vi "TransmissionAndAbsorptionSubVI.vi"(2 "FILTER":dbl[](array[numeric]), 3 "Stop REF":refnum<vi>, 4 "LED":dbl[](array[numeric])) -> (0 "Transmission":dbl[](array[numeric]), 1 "Absorption":dbl[](array[numeric]))   [LabVIEW 2021]
panel:
  in  "stop":bool
  in  "Array 2":dbl[](array[numeric])
  in  "Array":dbl[](array[numeric])
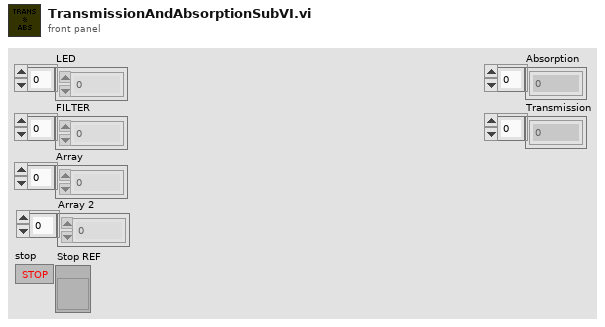
[diagram p1: front panel]
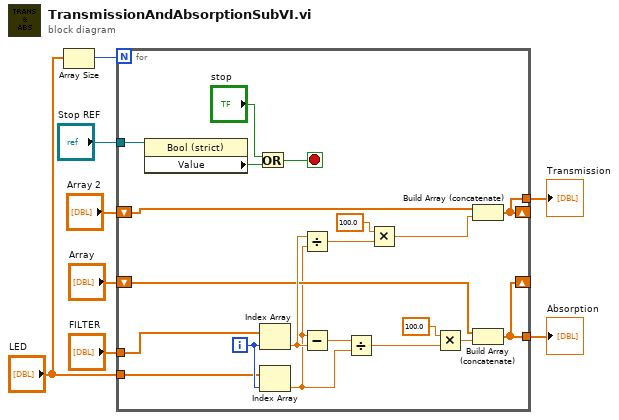
[diagram p0: block diagram]
diagram:
  n1 = Array Size(array="LED") -> (size(s)=w8:i32)
  n2 = for {
    N: w8 -> [_]
    tunnel: "LED" -> [w27]
    tunnel: "FILTER" -> [w26]
    shift-right: [w21] -> _
    shift-left: "Array 2" -> [w25]
    shift-right: [w22] -> _
    shift-left: "Array" -> [w23]
    tunnel: [w22] -> w5
    tunnel: [w21] -> w4
    tunnel: "Stop REF" -> [w16]
    i -> [w28]
    stop <- w17 stop-if-true
    n3 = property class="Bool (strict)"(reference=w16) -> ("Value"=w15:bool)  [unwired: 1 in, 2 out]
    n4 = Or(x="stop", y=w15) -> (x .or. y?=w17:bool)
    n5 = Index Array(array=w26, index=w28) -> (element=w24:dbl)
    n6 = Index Array(array=w27, index=w28) -> (element=w19:dbl)
    n7 = Divide(x=w24, y=w19) -> (x/y=w14:dbl)
    n8 = Subtract(x=w19, y=w24) -> (x-y=w20:dbl)
    n9 = Divide(x=w20, y=w19) -> (x/y=w12:dbl)
    n10 = Multiply(x=100.0, y=w14) -> (x*y=w10:dbl)
    n11 = Multiply(x=100.0, y=w12) -> (x*y=w9:dbl)
    n12 = Build Array (concatenate)(w25, w10) -> (w21:dbl[])
    n13 = Build Array (concatenate)(w23, w9) -> (w22:dbl[])
  }
  "Absorption" <- w5
  "Transmission" <- w4
